vi "FPGA_target_split_bit_information.vi"(1 "data in":u32 format="%01b") -> (0 "connector_data":T1)   [LabVIEW 2014]
doc: "splits a 32 bit number into a cluster of four bytes"
uses:
  FPGA_32BitPattern_data_type.ctl
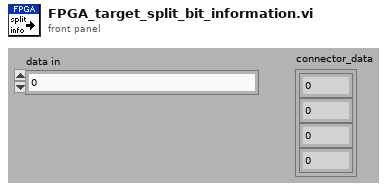
[diagram p1: front panel]
types:
  T1 = typedef "FPGA_32BitPattern_data_type.ctl" = cluster{"port0":u8, "port1":u8, "port2":u8, "port3":u8}
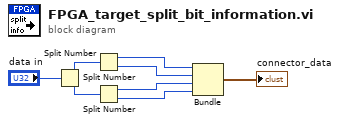
[diagram p0: block diagram]
diagram:
  n1 = Split Number(x="data in") -> (hi(x)=w7:u16, lo(x)=w6:u16)
  n2 = Split Number(x=w7) -> (hi(x)=w5:u8, lo(x)=w4:u8)
  n3 = Split Number(x=w6) -> (hi(x)=w3:u8, lo(x)=w2:u8)
  n4 = Bundle(w5, w4, w3, w2) -> (→"connector_data":cluster{u8, u8, u8, u8})  [unwired: 1 in]
